vi "Compute_OD.vi"(4 "timeout":u32=30000, 5 "params":T1, 6 "dark":u16[][](array[numeric]), 7 "flat":u16[][](array[numeric]), 8 "atoms":u16[][](array[numeric]), 9 "context in":refnum<class "zmq_context.lvclass">) -> (0 "error out":errorcluster, 1 "alpha":dbl, 2 "N":dbl, 3 "OD":sgl[][](array[numeric]))   [LabVIEW 2010]
uses:
  <vilib>/addons/zeromq/zmq_context.lvclass
panel:
  in  "error in":errorcluster
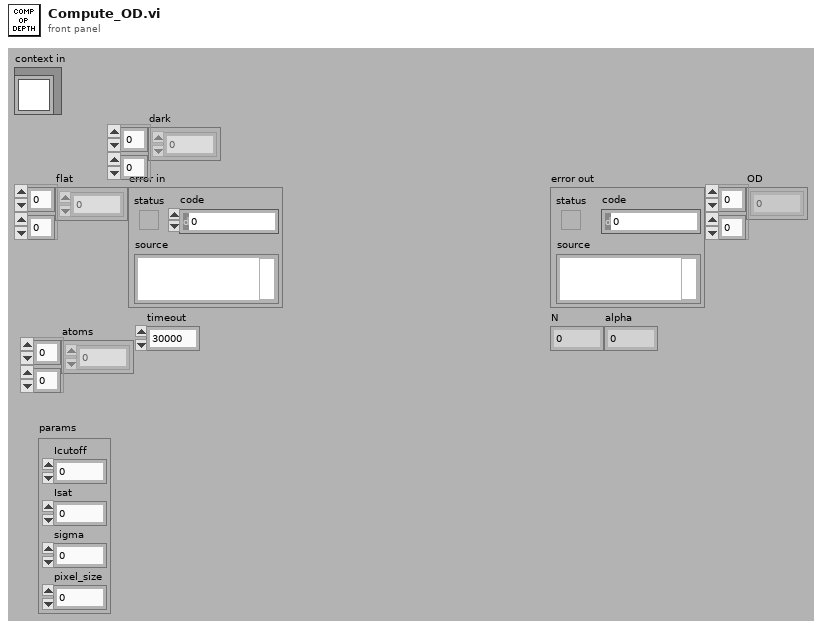
[diagram p1: front panel]
types:
  T1 = cluster{"Icutoff":dbl, "Isat":dbl, "sigma":dbl, "pixel_size":dbl}
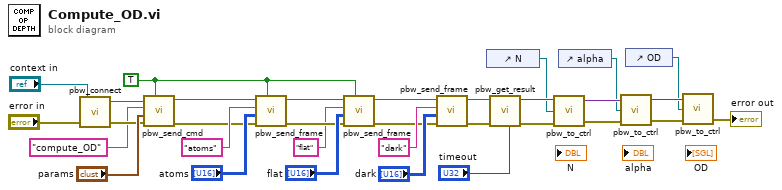
[diagram p0: block diagram]
diagram:
  w4 = TRUE ("more? (F)")
  n1 = call <vilib>:"pbw_connect.vi"("error in"="error in", "context in"="context in") -> ("error out"=w7:errorcluster, "socket out"=w6:refnum<class "zmq_socket.lvclass">)  [unwired: 2 in]
  n2 = call <vilib>:"pbw_send_cmd.vi"("more? (F)"=w4, "error in"=w7, "cluster"="params", "command"="compute_OD" ("data"), "socket in"=w6) -> ("error out"=w10:errorcluster, "socket out"=w11:refnum<class "zmq_socket.lvclass">)  [unwired: 2 in]
  n3 = call <vilib>:"pbw_send_frame.vi"("more? (F)"=w4, "error in"=w10, "data"="atoms", "name"="atoms", "socket in"=w11) -> ("error out"=w29:errorcluster, "socket out"=w30:refnum<class "zmq_socket.lvclass">)  [unwired: 2 in]
  n4 = call <vilib>:"pbw_send_frame.vi"("more? (F)"=w4, "error in"=w29, "data"="flat", "name"="flat", "socket in"=w30) -> ("error out"=w22:errorcluster, "socket out"=w23:refnum<class "zmq_socket.lvclass">)  [unwired: 2 in]
  n5 = call <vilib>:"pbw_send_frame.vi"("error in"=w22, "data"="dark", "name"="dark", "socket in"=w23) -> ("error out"=w2:errorcluster, "socket out"=w3:refnum<class "zmq_socket.lvclass">)  [unwired: 3 in]
  n6 = control-ref of="N"() -> (w15:refnum<vi>)
  n7 = call <vilib>:"pbw_get_result.vi"("error in"=w2, "socket in"=w3, "timeout"="timeout") -> ("error out"=w20:errorcluster, "return vals"=w21:variant)  [unwired: 4 in]
  n8 = call <vilib>:"pbw_to_ctrl.vi"("error in"=w20, "control"=w15, "variant w attribs"=w21) -> ("error out"=w16:errorcluster, "duplicate variant"=w17:variant)  [unwired: 1 out]
  n9 = control-ref of="alpha"() -> (w14:refnum<vi>)
  n10 = call <vilib>:"pbw_to_ctrl.vi"("error in"=w16, "control"=w14, "variant w attribs"=w17) -> ("error out"=w18:errorcluster, "duplicate variant"=w19:variant)  [unwired: 1 out]
  n11 = control-ref of="OD"() -> (w13:refnum<vi>)
  n12 = call <vilib>:"pbw_to_ctrl.vi"("error in"=w18, "control"=w13, "variant w attribs"=w19) -> ("error out"=→"error out":errorcluster)  [unwired: 2 out]
